vi "Read Voltage.vi"(8 "error in (no error)":errorcluster, 11 "Analog-Output in":refnum<class "Analog-Output.lvclass">) -> (0 "error out":errorcluster, 2 "Voltage":dbl, 3 "Analog-Output out":refnum<class "Analog-Output.lvclass">)   [LabVIEW 2019, in "Analog-Output.lvlib" / "Analog-Output.lvclass"]
uses:
  Library/Analog-Output.lvclass
  Library/Analog-Output.lvclass/Analog-Output.ctl
  Read Settings_All.vi
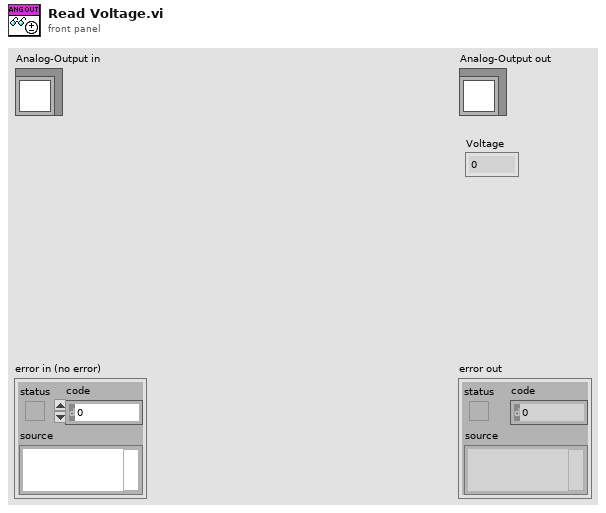
[diagram p1: front panel]
types:
  T1 = typedef "Analog-Output.lvlib/Analog-Output.lvclass/Settings.ctl" = cluster{"Voltage":dbl}
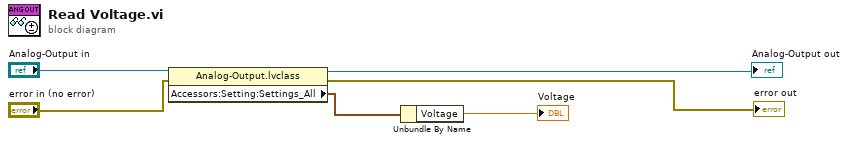
[diagram p0: block diagram]
diagram:
  n1 = property class="Analog-Output.lvclass"(reference="Analog-Output in", error in="error in (no error)") -> (reference out=→"Analog-Output out":refnum<class "Analog-Output.lvclass">, error out=→"error out":errorcluster, "Accessors:Setting:Settings_All"=w5:T1)
  n2 = Unbundle By Name(w5) -> ("Voltage"=→"Voltage":dbl)
